vi "GetListing.vi"(8 "error in (no error)":errorcluster, 10 "Server":path) -> (0 "error out":errorcluster, 1 "Found":bool, 3 "VI out":refnum<vi>)   [LabVIEW 2020]
panel:
  out "Array":T1(array[cluster])
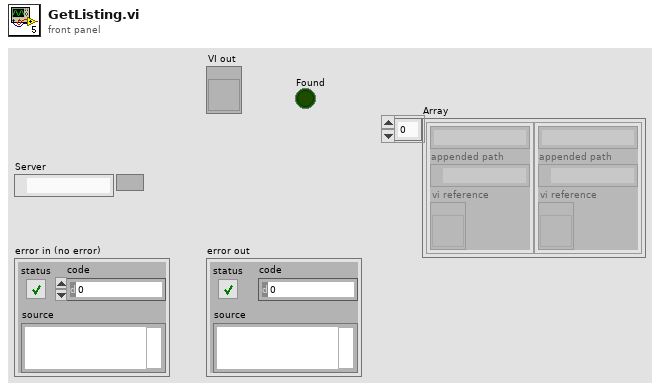
[diagram p1: front panel]
types:
  T1 = cluster{string, "appended path":path, "vi reference":refnum<vi>}[]
  T2 = cluster{string, "appended path":path, "vi reference":refnum<vi>}
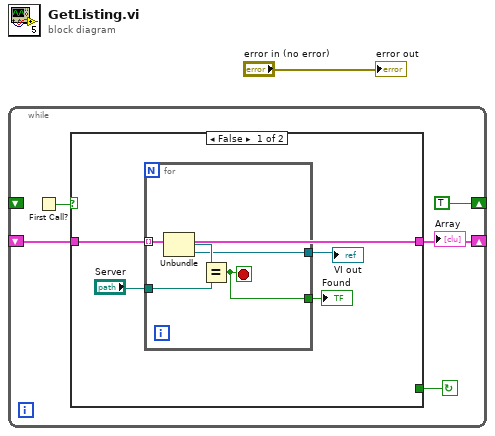
[diagram p0: block diagram]
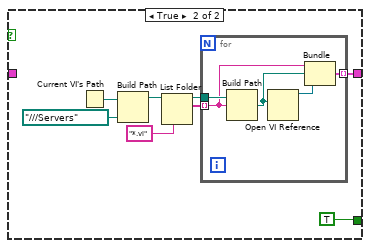
[diagram p2: hidden frame]
diagram:
  n1 = while {
    shift-right: [TRUE] -> _
    shift-left: _ -> [_]
    shift-right: [w5] -> _
    shift-left: _ -> [w4]
    stop <- w3 continue-if-true
    n2 = First Call?() -> (First Call?: T/F=w2:bool)
    n3 = case shown="False" w2 {
      tunnel: [w8 w17] -> w5
      tunnel: w4 -> [w8 _]
      tunnel: [_ TRUE] -> w3
      frame False {
        n4 = for {
          tunnel: w8 -> [w15] mode=indexing
          tunnel: "Server" -> [w13]
          tunnel: [w12] -> w9
          tunnel: [w11] -> w7
          stop <- w11 stop-if-true
          n5 = Unbundle(w15) -> ("appended path"=w14:path, "vi reference"=w12:refnum<vi>)  [unwired: 1 out]
          n6 = Equal?(x=w14, y=w13) -> (x = y?=w11:bool)
        }
        "VI out" <- w9
        "Found" <- w7
      }
      frame True {
        n7 = Current VI's Path() -> (path=w22:path)
        n8 = Build Path(base path=w22, name or relative path=path "../../../Servers") -> (appended path=w23:path)
        n9 = List Folder(path=w23, pattern="*.vi") -> (path out=w18:path, filenames=w19:string[])  [unwired: 2 in, 2 out]
        n10 = for {
          tunnel: w19 -> [w27] mode=indexing
          tunnel: w18 -> [w28]
          tunnel: [w24] -> w17 mode=indexing
          n11 = Build Path(base path=w28, name or relative path=w27) -> (appended path=w26:path)
          n12 = Open VI Reference(vi path=w26) -> (vi reference=w25:refnum<vi>)  [unwired: 5 in, 1 out]
          n13 = Bundle(w27, "appended path"=w26, "vi reference"=w25) -> (w24:T2)  [unwired: 1 in]
        }
      }
    }
    "Array" <- w5
  }
  "error out" <- "error in (no error)"
